vi "Get Status.vi"(0 "Notifier Name":string, 11 "Error In":errorcluster) -> (4 "Notifier Name DUP":string, 6 "Running?":bool, 8 "Current Frame":u32, 10 "Image Ref":T1, 15 "Error Out":errorcluster)   [LabVIEW 2020]
uses:
  <vilib>/vision/Image Controls.llb/IMAQ Image.ctl
  Hardware Configuration/Hardware Configuration Controls/Company.ctl
  Camera Controls/Camera IMAQ Key Info.ctl
  Hamamatsu/Orca Flash/Orca Flash Controls/Orca Flash Actions.ctl
  IDS/IDS Controls/IDS Actions.ctl
  Photometrics/Prime BSI/R Cubed SITK/Prime BSI R3 Controls/Prime R3 Actions.ctl
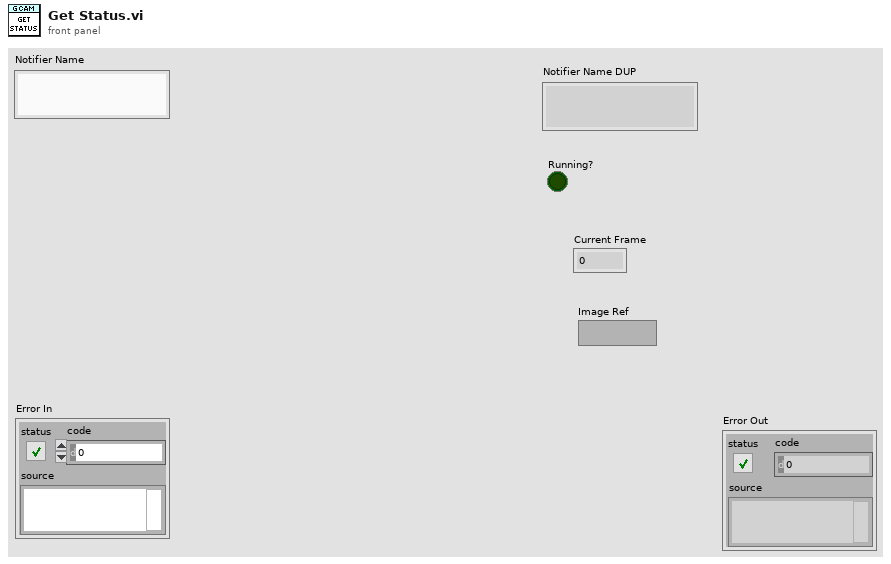
[diagram p1: front panel]
types:
  T1 = typedef "IMAQ Image.ctl" = refnum<image>
  T2 = typedef "Camera IMAQ Key Info.ctl" = cluster{"Frame":u32, "Sensor Height":i32, "Sensor Width":i32, "ROI Height":i32, "ROI Width":i32, "ROI Enable?":bool, "Bit per Pixel":u8}
  T3 = typedef "Company.ctl" = enum16{"AA Opto Electronic", "ASI", "Coherent", "Creset Optics", "CVI", "DAQmx", "Hamamatsu", "IDS", "Mad City Labs", "Marzhauser", "Measurement Computing", "MPB Com", "Olympus", "Photometrics", "PI", "Prior", "Thorlabs"}
  T4 = typedef "Orca Flash Actions.ctl" = enum16{"Idle", "Preview", "Record", "Record Settings", "Set Param", "Get Param", "Set ROI", "Get ROI", "Trigger Source", "Trigger Type", "Progessive Mode", "Area Mode", "Status", "Quit"}
  T5 = typedef "IDS Actions.ctl" = enum16{"Error Check", "Initialize", "Preview", "Record", "Abort", "Record Settings", "Set Parameter", "Get Parameter", "Set ROI", "Get ROI", "Status", "Quit"}
  T6 = typedef "Prime R3 Actions.ctl" = enum16{"Error Check", "Initialize", "Preview", "Record", "Abort", "Record Settings", "Set Parameter", "Get Parameter", "Set ROI", "Get ROI", "Status", "Set Trigger", "Quit"}
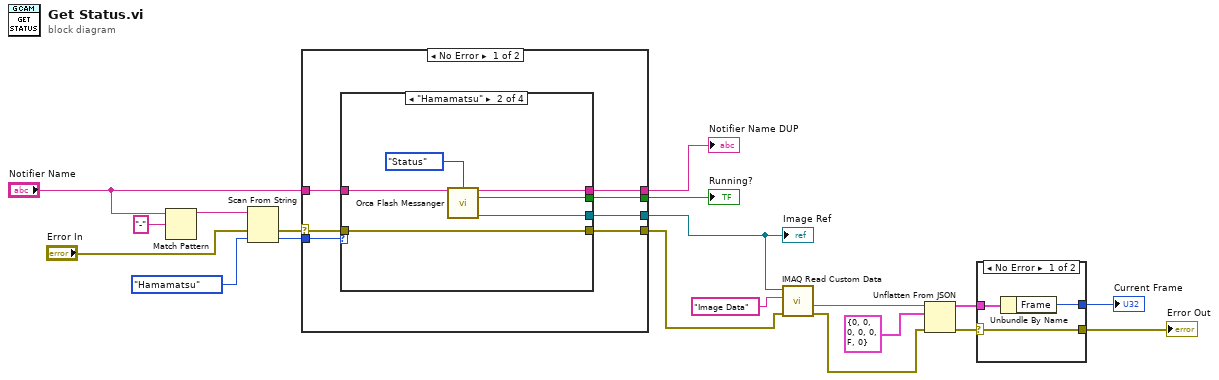
[diagram p0: block diagram]
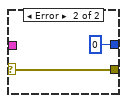
[diagram p2: hidden frame]
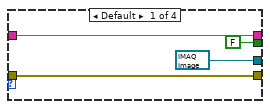
[diagram p3: hidden frame]
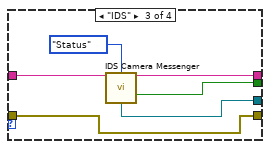
[diagram p4: hidden frame]
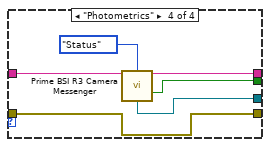
[diagram p5: hidden frame]
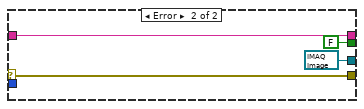
[diagram p6: hidden frame]
diagram:
  n1 = Match Pattern(string="Notifier Name", regular expression="-") -> (before substring=w17:string)  [unwired: 1 in, 3 out]
  n2 = Scan From String(input string=w17, error in="Error In", default 1=Company."Hamamatsu" ("Company")) -> (error out=w13:errorcluster, output 1=w16:T3)  [unwired: 2 in, 2 out]
  n3 = case shown="No Error" w13 {
    selector: w13 -> [w22 w51]
    tunnel: w16 -> [w26 _]
    tunnel: "Notifier Name" -> [w25 w52]
    tunnel: [w24 T1 refnum ("Image Ref")] -> w9
    tunnel: [w23 FALSE ("Running?")] -> w10
    tunnel: [w21 w52] -> w8
    tunnel: [w20 w51] -> w7
    frame No Error {
      n4 = case shown="\"Hamamatsu\"" w26 {
        tunnel: w25 -> [w30 w36 w42 w48]
        tunnel: [T1 refnum ("Image Ref") w35 w40 w45] -> w24
        tunnel: [FALSE ("Running?") w34 w38 w46] -> w23
        tunnel: w22 -> [w29 w32 w39 w44]
        tunnel: [w30 w33 w41 w47] -> w21
        tunnel: [w29 w32 w39 w44] -> w20
        frame Default {
        }
        frame "Hamamatsu" {
          n5 = call "Orca Flash Messanger.vi"("Notifier Name"=w36, "Camera Actions"=Orca_Flash_Actions."Status") -> ("Notifier Name Dup"=w33:string, "Running?"=w34:bool, "Image Ref"=w35:T1)  [unwired: 9 in, 2 out]
        }
        frame "IDS" {
          n6 = call "IDS Camera Messenger.vi"("Notifier Name"=w42, "IDS Actions"=IDS_Actions."Status") -> ("Notifier Name (Dup)"=w41:string, "Running?"=w38:bool, "Image Ref"=w40:T1)  [unwired: 8 in, 3 out]
        }
        frame "Photometrics" {
          n7 = call "Prime BSI R3 Camera Messenger.vi"("Notifier Name"=w48, "Prime Actions"=Prime_R3_Actions."Status") -> ("Notifier Name (Dup)"=w47:string, "Running?"=w46:bool, "Image Ref"=w45:T1)  [unwired: 8 in, 3 out]
        }
      }
    }
    frame Error {
    }
  }
  "Notifier Name DUP" <- w8
  "Image Ref" <- w9
  "Running?" <- w10
  n8 = call "IMAQ Read Custom Data"("error in (no error)"=w7, "Key"="Image Data", "Image"=w9) -> ("error out"=w3:errorcluster, "Custom Data Out"=w4:string)  [unwired: 6 in, 1 out]
  n9 = Unflatten From JSON(JSON string=w4, type and defaults=T2 {"Frame"=0, "Sensor Height"=0, "Sensor Width"=0, "ROI Height"=0, "ROI Width"=0, "ROI Enable?"=FALSE, "Bit per Pixel"=0} ("Camera IMAQ Key Info"), error in (no error)=w3) -> (value=w5:T2, error out=w2:errorcluster)  [unwired: 4 in]
  n10 = case shown="No Error" w2 {
    selector: w2 -> [w53 w56]
    tunnel: [w55 u32 0 ("Frame")] -> w11
    tunnel: w5 -> [w54 _]
    tunnel: [w53 w56] -> w1
    frame No Error {
      n11 = Unbundle By Name(w54) -> ("Frame"=w55:u32)
    }
    frame Error {
    }
  }
  "Error Out" <- w1
  "Current Frame" <- w11
